vi "Setpoint Status.vi"(8 "error in (no error)":errorcluster, 10 "Output (1:1)":u16(ring)=1 items=["1"=1, "2"=2, "3"=3, "4"=4], 11 "VISA resource name":refnum<visa-resource-name>) -> (0 "error out":errorcluster, 2 "Setpoint":dbl format="%.5f", 3 "VISA resource name out":refnum<visa-resource-name>)   [LabVIEW 2010, in "Lake Shore 350.lvlib"]
doc: "Returns the setpoint value for the selected output."
uses:
  <instrlib>/Lake Shore 350/Lake Shore 350.lvlib
  Instance           1 23Saved   Setpoint Status .vi
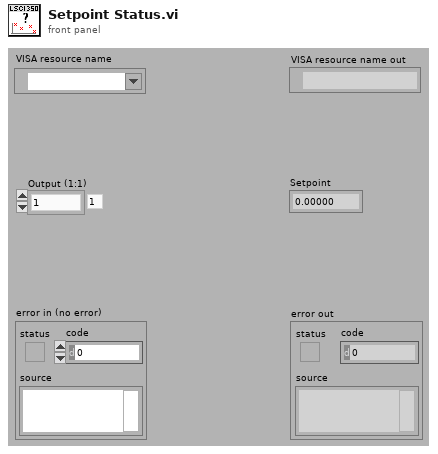
[diagram p1: front panel]
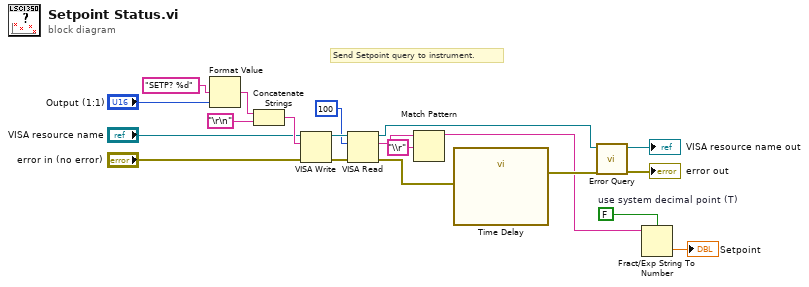
[diagram p0: block diagram]
diagram:
  w20 = FALSE  # use system decimal point (T)
  # "Send Setpoint query to instrument."
  n1 = Format Value(format string="SETP? %d", value (0)="Output (1:1)") -> (output string=w2:string)  [unwired: 1 in]
  n2 = Concatenate Strings(w2, "\r\n") -> (w11:string)
  n3 = VISA Write(VISA resource name="VISA resource name", write buffer=w11, error in (no error)="error in (no error)") -> (VISA resource name out=w15:refnum<visa-resource-name>, error out=w14:errorcluster)  [unwired: 1 out]
  n4 = VISA Read(VISA resource name=w15, byte count=100, error in (no error)=w14) -> (VISA resource name out=w7:refnum<visa-resource-name>, read buffer=w16:string, error out=w13:errorcluster)  [unwired: 1 out]
  n5 = Match Pattern(string=w16, regular expression="\\r") -> (before substring=w5:string)  [unwired: 1 in, 3 out]
  n6 = call "Time Delay"("error in (no error)"=w13) -> ("error out"=w8:errorcluster)  [unwired: 10 in]
  n7 = call <instrlib>:"Error Query.vi"("error in (no error)"=w8, "VISA resource name"=w7) -> ("error out"=→"error out":errorcluster, "VISA resource name out"=→"VISA resource name out":refnum<visa-resource-name>)  [unwired: 7 in, 1 out]
  n8 = Fract/Exp String To Number(use system decimal point (T)=w20, string=w5) -> (number=→"Setpoint":dbl)  [unwired: 2 in, 1 out]
